vi "SIM_FrameProperties.vi"(10 "file path (dialog if empty)":path) -> (0 "data":dbl[][](array[numeric]), 1 "Surf Loc (m)":dbl, 2 "Frame Properties (m)":T1, 3 "new file path (Not A Path if cancelled)":path)   [LabVIEW 2022 SP3]
uses:
  <vilib>/Utility/file.llb/Read Delimited Spreadsheet (DBL).vi
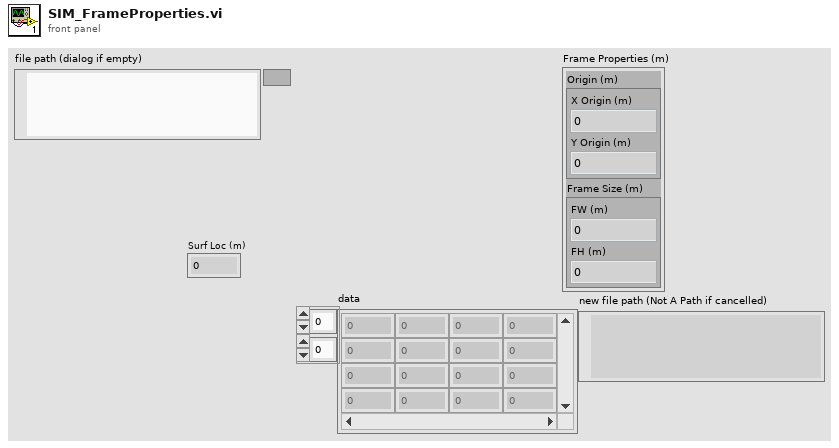
[diagram p1: front panel]
types:
  T1 = cluster{"Origin (m)":cluster{"X Origin (m)":dbl, "Y Origin (m)":dbl}, "Frame Size (m)":cluster{"FW (m)":dbl, "FH (m)":dbl}}
  T2 = cluster{"[0]":dbl, "[1]":dbl, "[2]":dbl, "[3]":dbl, "[4]":dbl, "[5]":dbl, "[6]":dbl, "[7]":dbl, "[8]":dbl}
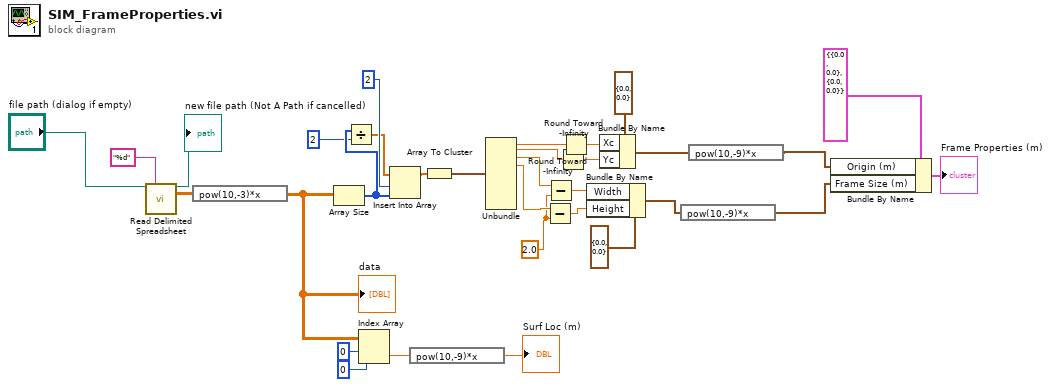
[diagram p0: block diagram]
diagram:
  w6 = 2.0 ("y")
  n1 = call-poly <vilib>:"Read Delimited Spreadsheet.vi"("file path (dialog if empty)"="file path (dialog if empty)", "format (%.3f)"="%d") -> ("new file path (Not A Path if cancelled)"=→"new file path (Not A Path if cancelled)":path, "all rows"=w27:dbl[][])  [unwired: 8 in, 4 out]
  n2 = expression code="pow(10,-3)*x"(w27) -> (w26:dbl[][])
  "data" <- w26
  n3 = Array Size(array=w26) -> (size(s)=w20:i32[])
  n4 = Divide(x=w20, y=2) -> (x/y=w21:dbl[])
  n5 = Index Array(array=w26, index (row)=0, index (col)=0 ("disabled index (col)")) -> (element=w24:dbl)
  n6 = Insert Into Array(array=w21, index=2, new element=w20) -> (w31:dbl[])
  n7 = expression code="pow(10,-9)*x"(w24) -> (→"Surf Loc (m)":dbl)
  n8 = Array To Cluster(array=w31) -> (cluster=w30:T2)
  n9 = Unbundle(w30) -> ("[0]"=w5:dbl, "[1]"=w2:dbl, "[2]"=w9:dbl, "[3]"=w7:dbl)  [unwired: 5 out]
  n10 = Subtract(x=w7, y=w6) -> (x-y=w8:dbl)
  n11 = Subtract(x=w9, y=w6) -> (x-y=w10:dbl)
  n12 = Round Toward -Infinity(1:w2) -> (0:w3:dbl)
  n13 = Round Toward -Infinity(1:w5) -> (0:w4:dbl)
  n14 = Bundle By Name(cluster=cluster{"Width":sgl, "Height":sgl} {"Width"=0.0, "Height"=0.0} ("Size (m)"), "Width"=w10, "Height"=w8) -> (w17:cluster{"Width":sgl, "Height":sgl})
  n15 = Bundle By Name(cluster=cluster{"Xc":sgl, "Yc":sgl} {"Xc"=0.0, "Yc"=0.0} ("Center coordinates (m)"), "Xc"=w4, "Yc"=w3) -> (w23:cluster{"Xc":sgl, "Yc":sgl})
  n16 = expression code="pow(10,-9)*x"(w17) -> (w13:cluster{"Width":sgl, "Height":sgl})
  n17 = expression code="pow(10,-9)*x"(w23) -> (w14:cluster{"Xc":sgl, "Yc":sgl})
  n18 = Bundle By Name(cluster=T1 {"Origin (m)"={"X Origin (m)"=0.0, "Y Origin (m)"=0.0}, "Frame Size (m)"={"FW (m)"=0.0, "FH (m)"=0.0}} ("Frame Properties (m)"), "Origin (m)"=w14, "Frame Size (m)"=w13) -> (→"Frame Properties (m)":T1)
